vi "RenameClassSpecific.vi"(0 "ClassWriterNative.lvclass":refnum<class "ClassWriterNative.lvclass">, 1 "ClassRef":refnum<vi>, 2 "NewClassPath":path, 5 "error in":errorcluster) -> (14 "ClassWriterNative.lvclass":refnum<class "ClassWriterNative.lvclass">, 19 "error out":errorcluster)   [LabVIEW 2020, in "ClassWriterNative.lvclass"]
uses:
  <resource>/Framework/Providers/Open_GDS/ClassProviders/Provider_LvNativeClass/ClassWriterNative_class/ClassWriterNative.lvclass
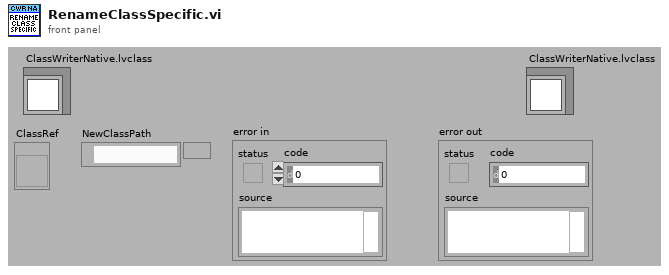
[diagram p1: front panel]
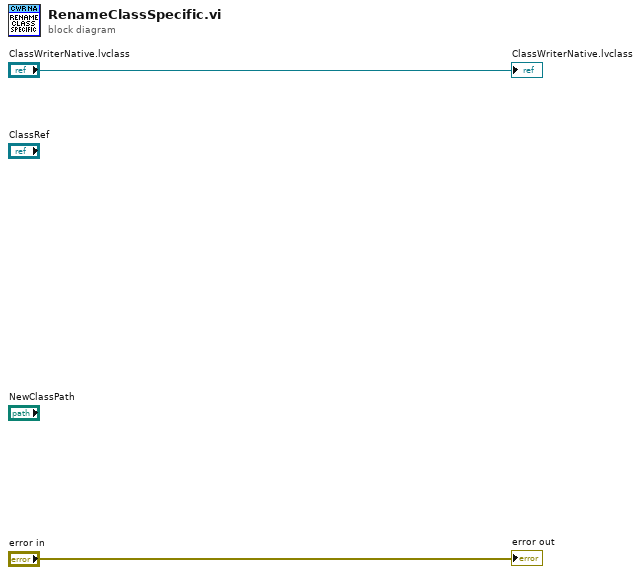
[diagram p0: block diagram]
diagram:
  "error out" <- "error in"
  "ClassWriterNative.lvclass" <- "ClassWriterNative.lvclass"
